vi "PointMap_Create.vi"(8 "error in (no error)":errorcluster, 10 "Name":string) -> (0 "error out":errorcluster, 3 "Map Out":T1)   [LabVIEW 2017, in "PointValueMap.lvlib"]
doc: "Creates a new map with the name you specify."
uses:
  <vilib>/addons/PointValueMap/PointValueMap.lvlib
  <vilib>/addons/PointValueMap/controls/PointMap.ctl
  <vilib>/addons/PointValueMap/controls/PointMapOperations.ctl
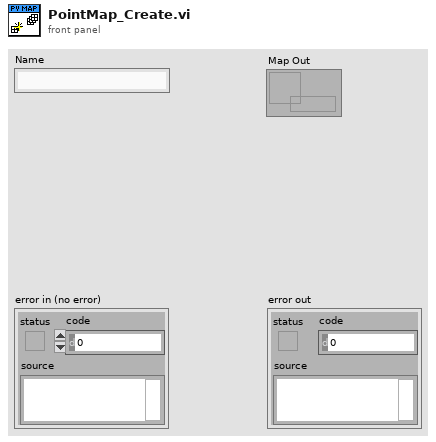
[diagram p1: front panel]
types:
  T1 = typedef "PointValueMap.lvlib/PointMap.ctl" = refnum<data-value>
  T2 = typedef "PointValueMap.lvlib/PointMapOperations.ctl" = enum16{"Initialize", "Create Map", "Update Map", "Get Map", "Get All Maps", "Destroy Map", "Destroy All Maps"}
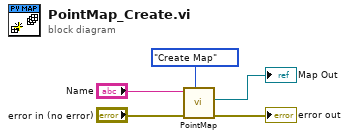
[diagram p0: block diagram]
diagram:
  n1 = call <vilib>:"PointMap.vi"("Operation"=PointMapOperations."Create Map", "error in (no error)"="error in (no error)", "Name"="Name") -> ("error out"=→"error out":errorcluster, "Map Out"=→"Map Out":T1)  [unwired: 4 in, 3 out]
